vi "initialise_controls.vi"(8 "error in (no error)":errorcluster, 11 "DL090216Display in":refnum<class "DisplayDL090216.lvclass">) -> (0 "error out":errorcluster, 3 "DL090216Display out":refnum<class "DisplayDL090216.lvclass">)   [LabVIEW 2010, in "DisplayDL090216.lvclass"]
uses:
  DisplayDL090216.lvclass
  DisplayDL090216.lvclass/DisplayDL090216.ctl
  common/classes/ErrorController/ErrorController/class_data.vi
  common/classes/ErrorController/ErrorController/ErrorController.lvclass
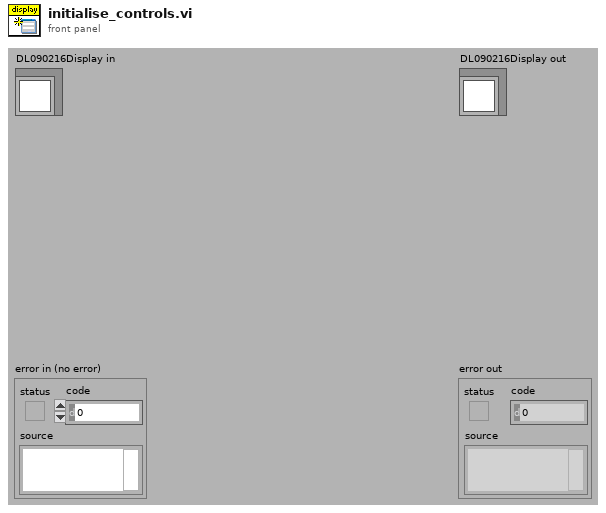
[diagram p1: front panel]
types:
  T1 = typedef "range_offset_cluster.ctl" = cluster{"range":dbl, "offset":dbl}
  T2 = typedef "channel_display_colour_enum.ctl" = enum16{"none", "red", "green", "blue", "grey scale", "custom"}
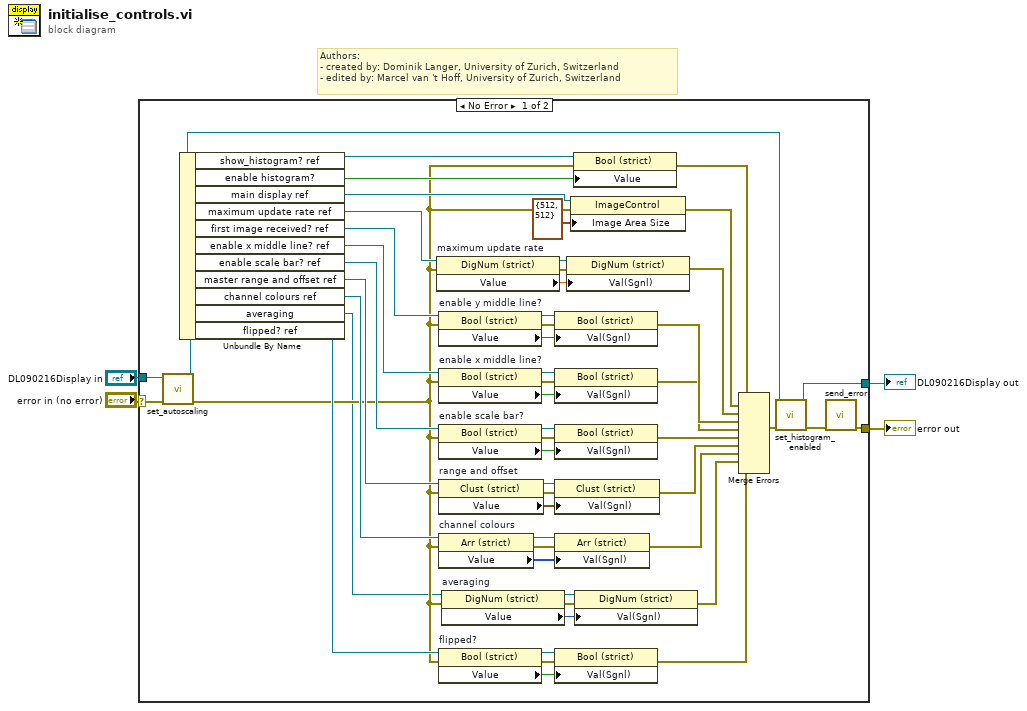
[diagram p0: block diagram]
diagram:
  # "Authors: \n- created by: Dominik Langer, University of Zurich, Switzerland\n- edited by: Marcel van 't Hoff, University of Zurich, Switzerland"
  n1 = case shown="No Error" "error in (no error)" {
    selector: "error in (no error)" -> [w26 w60]
    tunnel: [w28 w60] -> w4
    tunnel: [w24 w59] -> w2
    tunnel: "DL090216Display in" -> [w27 w59]
    frame No Error {
      n2 = call-dynamic "set_autoscaling.vi"("error in (no error)"=w26, "DisplayDL090216 in"=w27) -> ("error out"=w7:errorcluster, "DisplayDL090216 out"=w22:refnum<class "DisplayDL090216.lvclass">)  [unwired: 8 in]
      n3 = Unbundle By Name(w22) -> ("show_histogram? ref"=w23:refnum<vi>, "enable histogram?"=w21:bool, "main display ref"=w29:refnum<vi>, "maximum update rate ref"=w31:refnum<vi>, "first image received? ref"=w35:refnum<vi>, "enable x middle line? ref"=w36:refnum<vi>, "enable scale bar? ref"=w46:refnum<vi>, "master range and offset ref"=w47:refnum<vi>, "channel colours ref"=w52:refnum<vi>, "averaging"=w6:refnum<vi>, "flipped? ref"=w56:refnum<vi>)
      n4 = property on="maximum update rate" class="DigNum (strict)"(reference=w31, error in=w7) -> (reference out=w32:refnum<vi>, error out=w33:errorcluster, "Value"=w34:dbl[unit])
      n5 = property on="enable y middle line?" class="Bool (strict)"(reference=w35, error in=w7) -> (reference out=w39:refnum<vi>, error out=w38:errorcluster, "Value"=w37:bool)
      n6 = property on="enable x middle line?" class="Bool (strict)"(reference=w36, error in=w7) -> (reference out=w40:refnum<vi>, error out=w41:errorcluster, "Value"=w42:bool)
      n7 = property on="enable scale bar?" class="Bool (strict)"(reference=w46, error in=w7) -> (reference out=w45:refnum<vi>, error out=w44:errorcluster, "Value"=w43:bool)
      n8 = property on="range and offset" class="Clust (strict)"(reference=w47, error in=w7) -> (reference out=w49:refnum<vi>, error out=w50:errorcluster, "Value"=w48:T1)
      n9 = property on="channel colours" class="Arr (strict)"(reference=w52, error in=w7) -> (reference out=w53:refnum<vi>, error out=w54:errorcluster, "Value"=w51:T2[])
      n10 = property on="flipped?" class="Bool (strict)"(reference=w56, error in=w7) -> (reference out=w55:refnum<vi>, error out=w57:errorcluster, "Value"=w58:bool)
      n11 = property on="averaging" class="DigNum (strict)"(reference=w6, error in=w7) -> (reference out=w5:refnum<vi>, error out=w9:errorcluster, "Value"=w10:i32)
      n12 = property on="Property Node" class="Bool (strict)"(reference=w39, error in=w38, "Val(Sgnl)"=w37) -> (error out=w20:errorcluster)  [unwired: 1 out]
      n13 = property on="Property Node" class="Bool (strict)"(reference=w40, error in=w41, "Val(Sgnl)"=w42) -> (error out=w19:errorcluster)  [unwired: 1 out]
      n14 = property on="Property Node" class="Bool (strict)"(reference=w45, error in=w44, "Val(Sgnl)"=w43) -> (error out=w18:errorcluster)  [unwired: 1 out]
      n15 = property on="Property Node" class="Clust (strict)"(reference=w49, error in=w50, "Val(Sgnl)"=w48) -> (error out=w17:errorcluster)  [unwired: 1 out]
      n16 = property on="Property Node" class="Arr (strict)"(reference=w53, error in=w54, "Val(Sgnl)"=w51) -> (error out=w16:errorcluster)  [unwired: 1 out]
      n17 = property on="Property Node" class="Bool (strict)"(reference=w55, error in=w57, "Val(Sgnl)"=w58) -> (error out=w15:errorcluster)  [unwired: 1 out]
      n18 = property on="Property Node" class="DigNum (strict)"(reference=w32, error in=w33, "Val(Sgnl)"=w34) -> (error out=w14:errorcluster)  [unwired: 1 out]
      n19 = property on="Property Node" class="ImageControl"(reference=w29, error in=w7, "Image Area Size"=cluster{"Width":u32, "Height":u32} {"Width"=512, "Height"=512} ("Image Area:Size:All Elements")) -> (error out=w13:errorcluster)  [unwired: 1 out]
      n20 = property on="Property Node" class="Bool (strict)"(reference=w23, error in=w7, "Value"=w21) -> (error out=w12:errorcluster)  [unwired: 1 out]
      n21 = property on="Property Node" class="DigNum (strict)"(reference=w5, error in=w9, "Val(Sgnl)"=w10) -> (error out=w8:errorcluster)  [unwired: 1 out]
      n22 = Merge Errors(w12, w13, w14, w20, w19, w18, w17, w16, w8, w15) -> (w11:errorcluster)
      n23 = call-dynamic "set_histogram_enabled.vi"("error in (no error)"=w11, "DisplayDL090216 in"=w22) -> ("error out"=w25:errorcluster, "DisplayDL090216 out"=w24:refnum<class "DisplayDL090216.lvclass">)  [unwired: 8 in]
      n24 = call "send_error.vi"("error in (no error)"=w25) -> ("error out"=w28:errorcluster)  [unwired: 10 in]
    }
    frame Error {
    }
  }
  "error out" <- w4
  "DL090216Display out" <- w2
